vi "Experiment header-Calculate STATS.vi"(10 "Logging queue element":T1={"Imaging Protocol"=enum."Live Imaging", "Number of Trials"=0, "Frame Size"=100, "# Averaged frames"=0, "Dwell time (us)"=0.1, "Index of Z-plane"=0, "Timelapse?"=FALSE, "Logging process is active"=FALSE, "Speed logging enabled"=FALSE, "tdms file ref"=refnum, "path"=path "", "Trial Number"=0, "Expected # points acquired"=FALSE, "Manually stopped"=FALSE, "Ch0 data"=[], "Ch1 data"=[], "Last trial"=FALSE, "Points acquired"={"Ch0 last trial"=0, "Ch1 last trial"=0, "All trials"=0}} {"Frame Size" items=["100X100"=100, "128X128"=128, "200X200"=200, "256X256"=256, "512X512"=512, "1024x1024"=1024, "2048x2048"=2048]; "Dwell time (us)" format="%#.6g"}, 11 "Timelapse frames saved":u32) -> (1 "Number of acquired frames":dbl, 2 "Acquisition time (ms)":dbl format="%#_9f", 3 "Total number of points acquired (Ch0)":dbl)   [LabVIEW 2013]
uses:
  Typedefs/Logging queue element.ctl
  Typedefs/Imaging Protocols enum.ctl
  Typedefs/Frame Size.ctl
  Typedefs/Acquired points count.ctl
  Typedefs/Save-Load-Save as-Load last enum.ctl
  Typedefs/Header file type enum.ctl
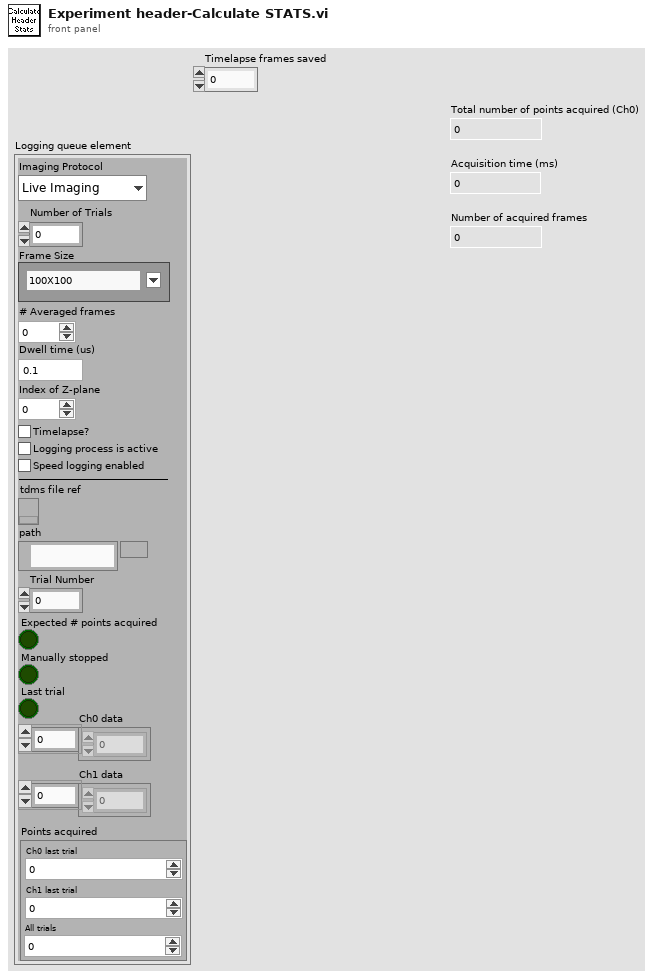
[diagram p1: front panel]
types:
  T1 = typedef "Logging queue element.ctl" = cluster{"Imaging Protocol":T2, "Number of Trials":u16, "Frame Size":T3, "# Averaged frames":u16, "Dwell time (us)":dbl, "Index of Z-plane":i32, "Timelapse?":bool, "Logging process is active":bool, "Speed logging enabled":bool, "tdms file ref":refnum<k34>, "path":path, "Trial Number":i32, "Expected # points acquired":bool, "Manually stopped":bool, "Ch0 data":u32[], "Ch1 data":u32[], "Last trial":bool, "Points acquired":T4}
  T2 = typedef "Imaging Protocols enum.ctl" = enum16{"AOL Z-Stack", "Motor Z Stack", "Functional Acquisition", "Single Plane Acquisition", "Volume Acquisition", "Live Imaging", "Live Plane Imaging", "Live Volume Imaging"}
  T3 = typedef "Frame Size.ctl" = u16
  T4 = typedef "Acquired points count.ctl" = cluster{"Ch0 last trial":u64, "Ch1 last trial":u64, "All trials":u64}
  T5 = typedef "Header file type enum.ctl" = enum16{"All parameters", "Params for funct acq w ROI or mscn", "Params for funct acq w rectangles", "Live imaging header parameters", "AOL Parameters"}
  T6 = typedef "Save-Load-Save as-Load last enum.ctl" = enum16{"Save file", "Save file as", "Load file", "Load last file"}
  T7 = typedef "AOL_Globals.ctl" = cluster{"Imaging Protocol":T2, "Number of POI":u16, "Number of Miniscans":u16, "Number of Trials":u16, "Number of Cycles ":u64, "# Averaged Frames":u16, "Laser power (%)":u8, "Pockels":dbl, "Acquisition Length (sec)":dbl, "Fill time (us)":dbl, "POI Dwell time (us)":dbl, "Miniscan Dwell time per pixel (us)":dbl, "PMT 1":dbl, "PMT 2":dbl, "Back Apperture":dbl, "Frame Size":T3, "Center Frequency":dbl, "Field of View":dbl, "DwellTime (us)":dbl, "Wavelength (nm)":dbl, "Zoom":dbl, "AOL Z":dbl, "AOL Mode":T8, "GridXY":dbl, "GridZ":dbl, "TriggerPeriod (sec)":dbl, "Number of Pixels in Miniscan":u16, "Experiment folder path":path, "X centre":dbl, "Y centre":dbl, "Angle (degrees)":dbl, "Plane Mode":T9, "Threshold":u16[], "Regenerate Chirps":bool, "Rectangle ROI length (pixels)":u16, "Rectangle ROI height (pixels)":u16, "AOD fill":u16, "Samples Wait after Trigger":u16, "StartUp Delay":i32, "Slip Cycle":u32, "Add Cycle":bool}
  T8 = typedef "AOL modes.ctl" = enum16{"Raster", "Structural", "Pointing", "Mini Scan", "Alignment"}
  T9 = typedef "Plane Mode.ctl" = u16
  T10 = typedef "Header parameters cluster-ALL.ctl" = cluster{"Imaging Protocol":T2, "Number of POI":u16, "Number of Miniscans":u16, "Number of Trials":u16, "Number of Cycles ":u64, "# Averaged Frames":u16, "Laser power (%)":u8, "Pockels":dbl, "Acquisition Length (sec)":dbl, "Fill time (us)":dbl, "POI Dwell time (us)":dbl, "Miniscan Dwell time per pixel (us)":dbl, "PMT 1":dbl, "PMT 2":dbl, "Back Apperture":dbl, "Zoom":dbl, "Frame Size":T3, "Center Frequency":dbl, "Field of View":dbl, "DwellTime (us)":dbl, "Wavelength (nm)":dbl, "AOL Z":dbl, "AOL Mode":T8, "GridXY":dbl, "GridZ":dbl, "TriggerDelay (sec)":dbl, "Number of Pixels in Miniscan":u16, "Experiment folder path":path, "X centre":dbl, "Y centre":dbl, "Angle (degrees)":dbl, "Plane Mode":T9, "Software version":dbl, "Objective":T11, "MotorZ Calibration":u32, "Pockels Calibration":u32, "Threshold":u16[], "Video length (sec)":dbl, "Frame rate (fps)":u8, "Rectangle ROI length (pixels)":u16, "Rectangle ROI height (pixels)":u16}
  T11 = typedef "Objective selector control enum.ctl" = string
  T12 = typedef "ROI parameters data type.ctl" = cluster{"ROI index":dbl, "ROI ID":dbl, "ROI Time (ns)":dbl, "Pixels in ROI":dbl, "X start":dbl, "Y start":dbl, "Z start":dbl, "X stop":dbl, "Y stop":dbl, "Z stop":dbl, "Angle (deg)":dbl, "Composite ID":dbl, "Number of lines":dbl, "Frame Size":dbl, "Zoom":dbl, "Laser Power (%)":dbl, "ROI group ID":dbl}
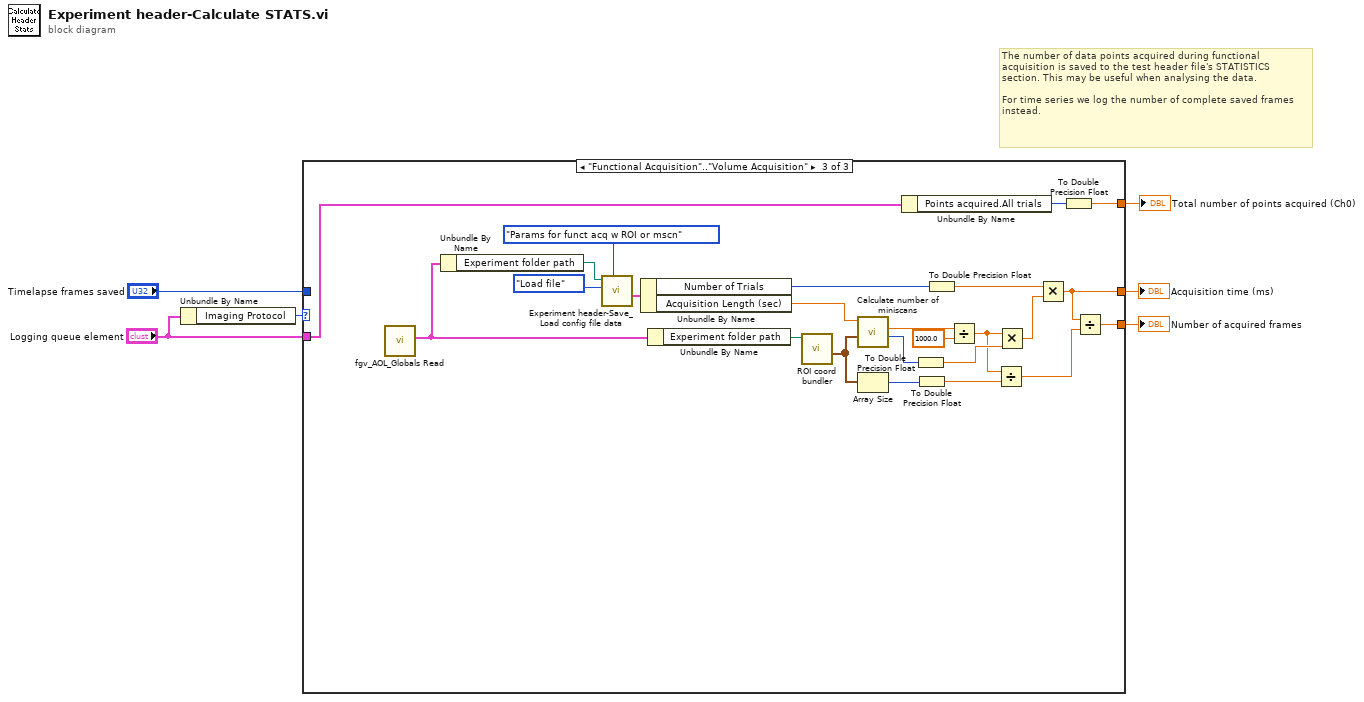
[diagram p0: block diagram]
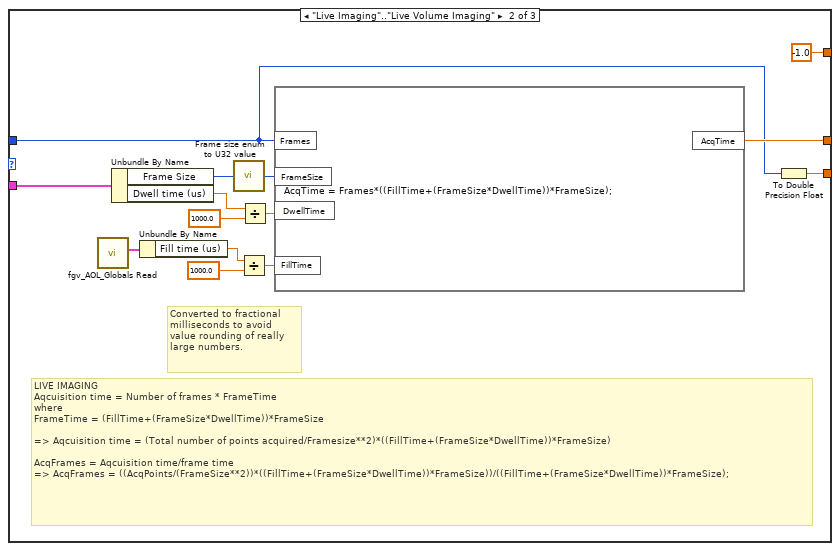
[diagram p3: hidden frame]
diagram:
  # "The number of data points acquired during functional acquisition is saved to the test header file's STATISTICS section. This may be useful when analysing the data.\n\nFor time series we log the number of complete saved frames instead."
  n1 = Unbundle By Name("Logging queue element") -> ("Imaging Protocol"=w6:T2)
  n2 = case shown="\"Functional Acquisition\"..\"Volume Acquisition\"" w6 {
    tunnel: [_ w20 w29] -> w5
    tunnel: [_ w8 w27] -> w4
    tunnel: "Logging queue element" -> [_ w10 w22]
    tunnel: [_ -1.0 ("Ch0") w21] -> w2
    tunnel: "Timelapse frames saved" -> [_ w7 _]
    frame "AOL Z-Stack", "Motor Z Stack" {
    }
    frame "Live Imaging".."Live Volume Imaging" {
      # "LIVE IMAGING\nAqcuisition time = Number of frames * FrameTime\nwhere\nFrameTime = (FillTime+(FrameSize*DwellTime))*FrameSize\n\n=> Aqcuisition time = (Total number of points acquired/Framesize**2)*((FillTime+(FrameSize*DwellTime))*FrameSize)\n\nAcqFrames = Aqcuisition time/frame time\n=> AcqFrames = ((AcqPoints/(FrameSize**2))*((FillTime+(FrameSize*DwellTime))*FrameSize))/((FillTime+(FrameSize*DwellTime))*FrameSize);"
      # "Converted to fractional milliseconds to avoid value rounding of really large numbers."
      n3 = call "fgv_AOL_Globals Read.vi"() -> ("AOL_Globals"=w15:T7)  [unwired: 9 in, 2 out]
      n4 = Unbundle By Name(w10) -> ("Frame Size"=w12:T3, "Dwell time (us)"=w11:dbl)
      n5 = Unbundle By Name(w15) -> ("Fill time (us)"=w18:dbl)
      n6 = call "Frame size enum to U32 value.vi"("Value"=w12) -> ("Frame Size U32"=w19:u32)
      n7 = Divide(x=w18, y=1000.0) -> (x/y=w14:dbl)
      n8 = Divide(x=w11, y=1000.0) -> (x/y=w13:dbl)
      n9 = formula code="AcqTime = Frames*((FillTime+(FrameSize*DwellTime))*FrameSize);"("FrameSize"=w19, "DwellTime"=w13, "FillTime"=w14, "Frames"=w7) -> ("AcqTime"=w20:dbl)
      n10 = To Double Precision Float(number=w7) -> (double precision float=w8:dbl)
    }
    frame "Functional Acquisition".."Volume Acquisition" {
      n11 = call "fgv_AOL_Globals Read.vi"() -> ("AOL_Globals"=w38:T7)  [unwired: 9 in, 2 out]
      n12 = Unbundle By Name(w38) -> ("Experiment folder path"=w40:path)
      n13 = call "Experiment header-Save_Load config file data.vi"("Header file type"=Header_file_type_enum."Params for funct acq w ROI or mscn", "Function"=Save-Load-Save_as-Load_last_enum."Load file", "Experiment data folder path"=w40) -> ("All header parameters out"=w42:T10)  [unwired: 7 in, 1 out]
      n14 = Unbundle By Name(w42) -> ("Number of Trials"=w32:u16, "Acquisition Length (sec)"=w43:dbl)
      n15 = Unbundle By Name(w38) -> ("Experiment folder path"=w39:path)
      n16 = call "ROI coord bundler.vi"("Experiment folder path"=w39) -> ("ROI Attributes"=w30:T12[])  [unwired: 3 in, 7 out]
      n17 = call "Calculate number of miniscans.vi"("XYZ Coordinates"=w30, "Acquisition length (sec)"=w43) -> ("Number of cycles"=w35:u64, "Cycle time (us)"=w37:dbl)  [unwired: 7 in, 1 out]
      n18 = Array Size(array=w30) -> (size(s)=w28:i32)
      n19 = Unbundle By Name(w22) -> ("Points acquired.All trials"=w23:u64)
      n20 = To Double Precision Float(number=w35) -> (double precision float=w34:dbl)
      n21 = To Double Precision Float(number=w28) -> (double precision float=w25:dbl)
      n22 = To Double Precision Float(number=w32) -> (double precision float=w31:dbl)
      n23 = Divide(x=w37, y=1000.0) -> (x/y=w26:dbl)
      n24 = Divide(x=w26, y=w25) -> (x/y=w24:dbl)
      n25 = Multiply(x=w26, y=w34) -> (x*y=w33:dbl)
      n26 = Multiply(x=w31, y=w33) -> (x*y=w29:dbl)
      n27 = To Double Precision Float(number=w23) -> (double precision float=w21:dbl)
      n28 = Divide(x=w29, y=w24) -> (x/y=w27:dbl)
    }
  }
  "Total number of points acquired (Ch0)" <- w2
  "Number of acquired frames" <- w4
  "Acquisition time (ms)" <- w5
